vi "Gas Auswahl aus Komponenten.vi"(8 "Fehler (Eingang, kein Fehler)":errorcluster, 10 "Gasnummer:":u8, 11 "Komponentenauswahl":T1 {"Konzentration" format="%#.6f"}) -> (0 "Fehler (Ausgang)":errorcluster, 2 "Konzentration":dbl, 3 "Auswahl":T2)   [LabVIEW 2020, in "Linearisierung v2.lvlib"]
uses:
  Linearisierung v2.lvlib
  Visualisierungs Elemente/Auswahlfeld.ctl
  KomponentenArray.ctl
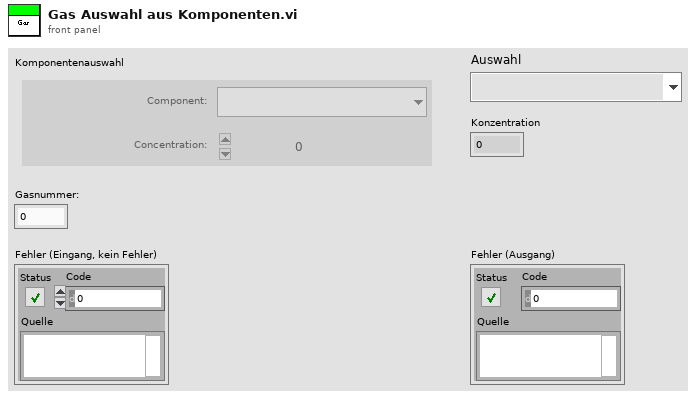
[diagram p1: front panel]
types:
  T1 = typedef "Linearisierung v2.lvlib/KomponentenArray.ctl" = cluster{"Komponente:":T2, "Konzentration":dbl}[]
  T2 = typedef "Auswahlfeld.ctl" = u16
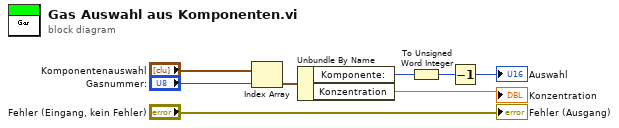
[diagram p0: block diagram]
diagram:
  n1 = Index Array(array="Komponentenauswahl", index="Gasnummer:") -> (element=w3:cluster{"Komponente:":T2, "Konzentration":dbl})
  n2 = Unbundle By Name(w3) -> ("Komponente:"=w4:T2, "Konzentration"=→"Konzentration":dbl)
  n3 = To Unsigned Word Integer(number=w4) -> (unsigned 16bit integer=w6:T2)
  n4 = Decrement(x=w6) -> (x-1=→"Auswahl":T2)
  "Fehler (Ausgang)" <- "Fehler (Eingang, kein Fehler)"
